vi "XY stage Buttons (reduced).vi"() -> ()   [LabVIEW 2017]
panel:
  in  "Move Inverse":bool
  in  "Move Normal":bool
  out "Expected Output":cluster{"X":dbl, "Y":dbl}[](graph)
  out "Total Time Horizontal":dbl
  out "Total Time Vertical":dbl
  in  "Velocity and Acceleration of Absolute":cluster{"Velocity":dbl, "Acceleration":dbl}={"Velocity"=150.0, "Acceleration"=2000.0} {"Acceleration" min=0.0; "Velocity" min=0.0}
  in  "Abort Motion":bool
  out "Total Y Path":dbl
  in  "Absolute Movement 2":cluster{"X Position":dbl, "Y Position":dbl}[](array[cluster]) {"Y Position" min=-100.0 max=100.0; "X Position" min=-100.0 max=100.0}
  in  "Start Absolute 2":bool
  out "Current Y Position":dbl[](array[numeric])
  out "Current X Position":dbl[](array[numeric])
  out "Total X Path":dbl
  in  "Number of Horizontal Segments":u32
  in  "Number of Vertical Segments":u32
  in  "Horizontal Segments Parameters":T1(array[cluster]) {"velocity" min=0.0; "Y rel dist" min=-100.0 max=100.0; "X rel dist" min=-100.0 max=100.0}
  in  "Vertical Segments Parameters":T1(array[cluster]) {"velocity" min=0.0; "Y rel dist" min=-100.0 max=100.0; "X rel dist" min=-100.0 max=100.0}
  in  "Absolute Movement 1":cluster{"X Position":dbl, "Y Position":dbl}[](array[cluster]) {"Y Position" min=-100.0 max=100.0; "X Position" min=-100.0 max=100.0}
  in  "Start Absolute 1":bool
  in  "Go Home":bool
  in  "Kill All":bool
  # "Relative Movement"
  # "Absolute Movement"
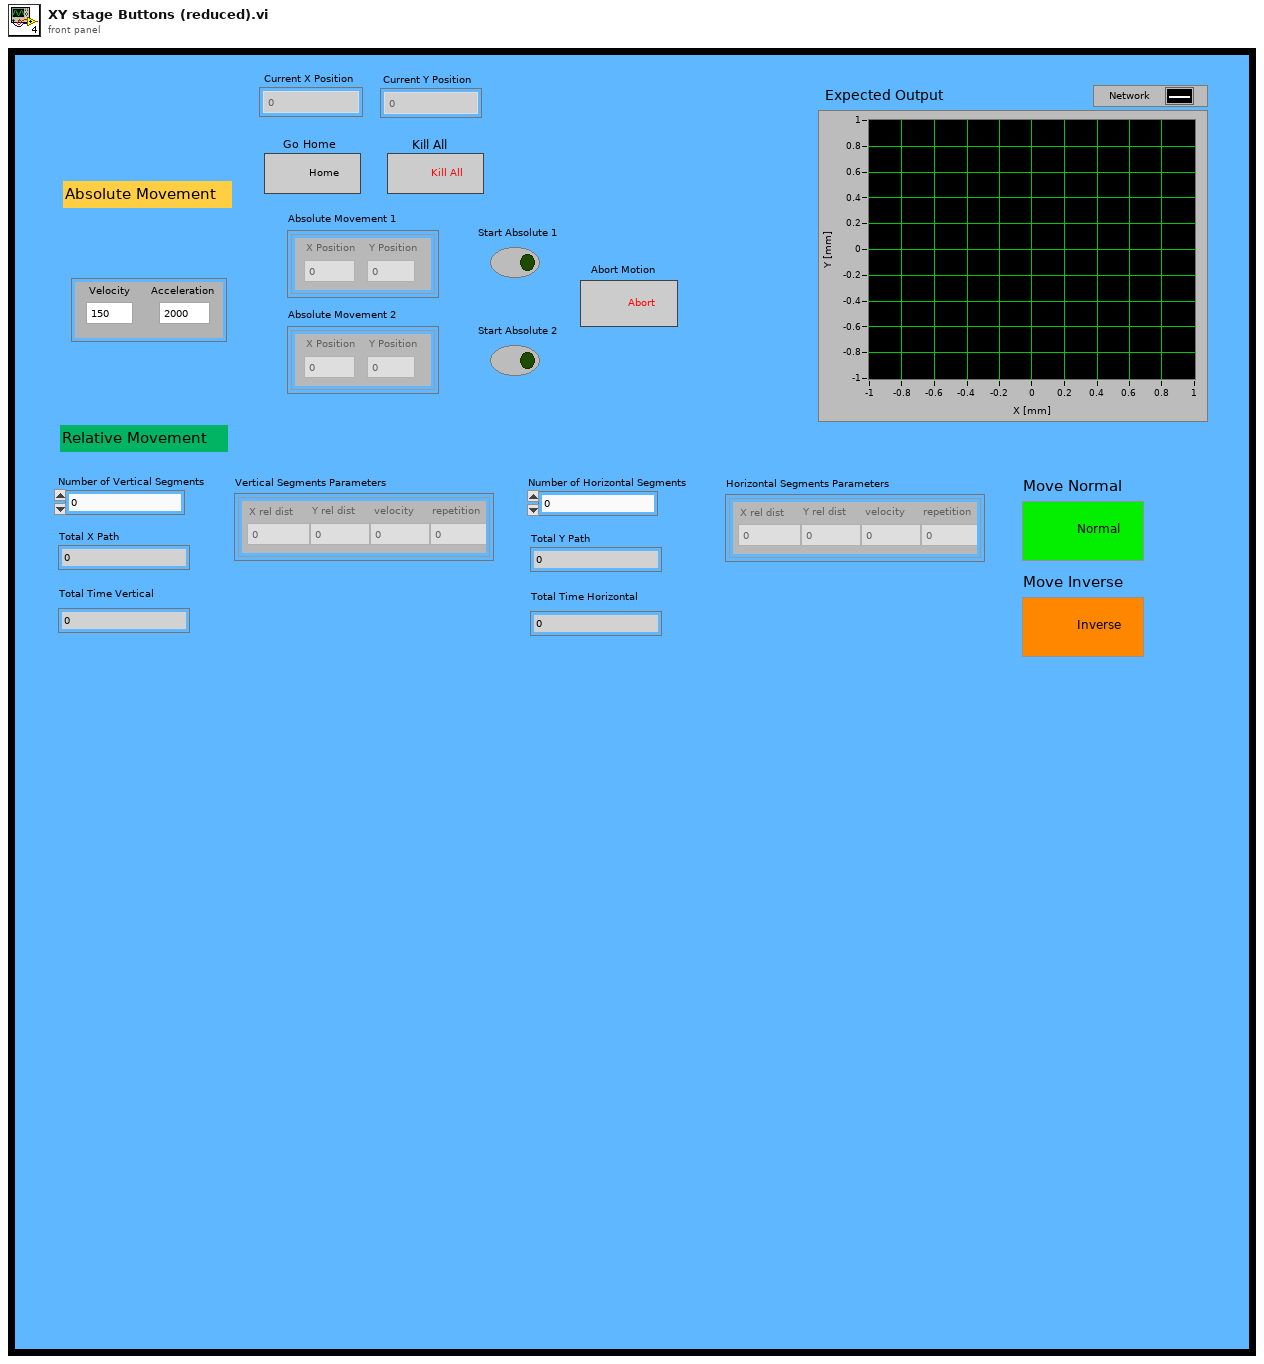
[diagram p1: front panel]
types:
  T1 = cluster{"X rel dist":dbl, "Y rel dist":dbl, "velocity":dbl, "repetition":u32}[]
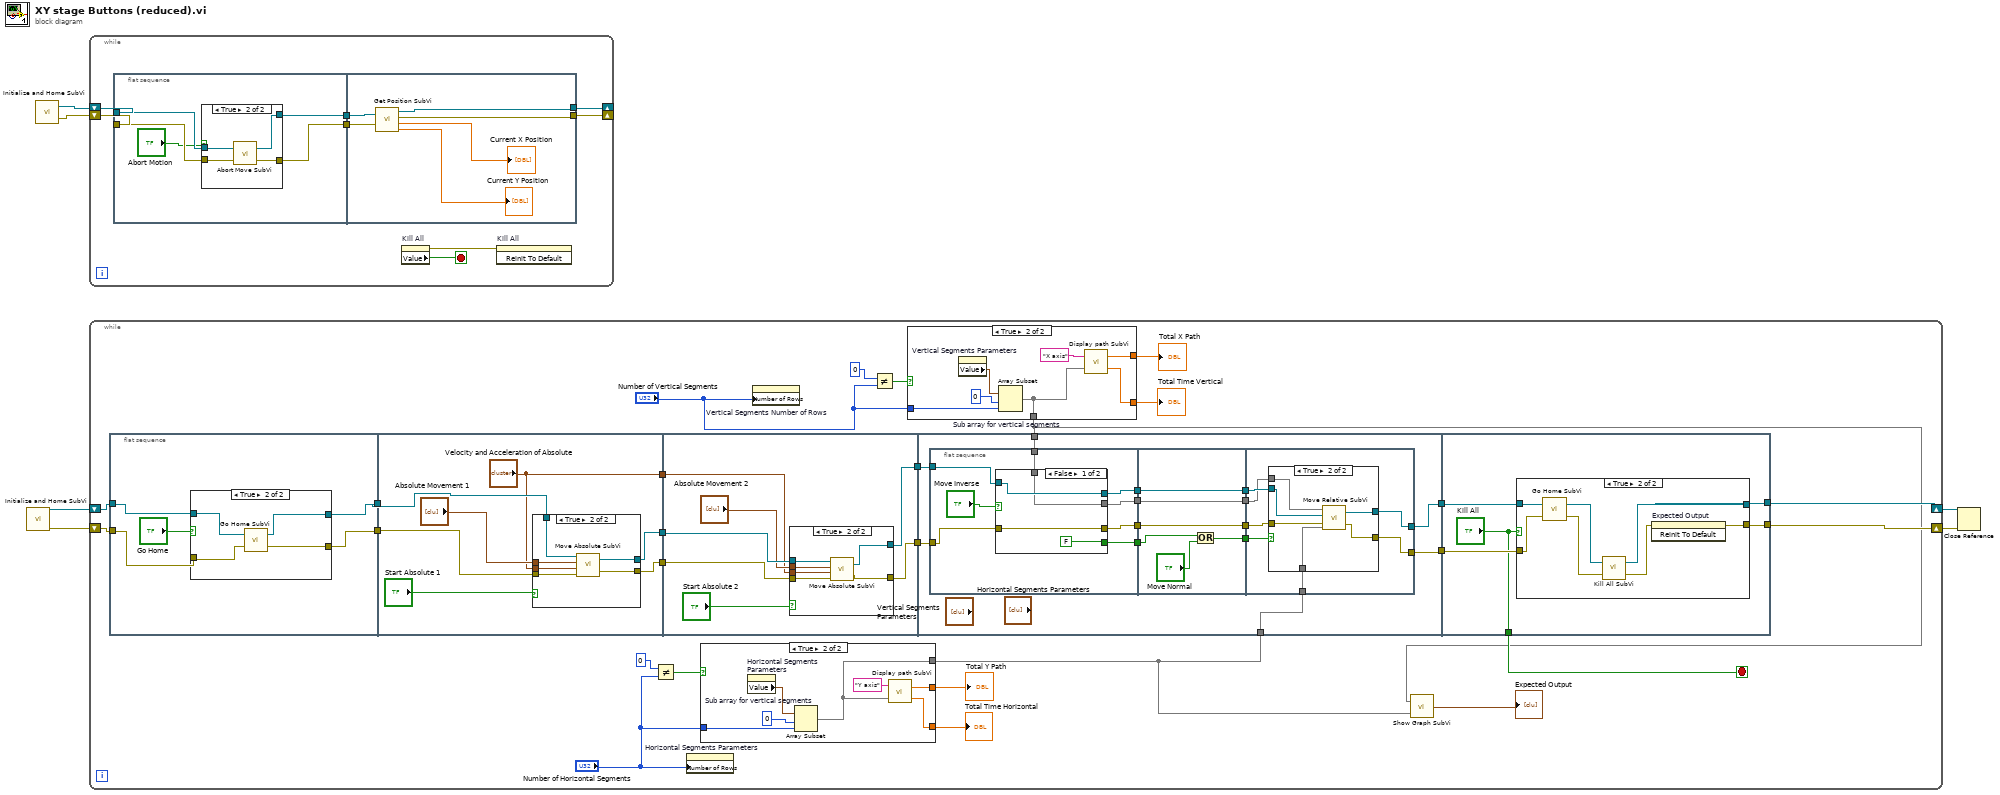
[diagram p0: block diagram]
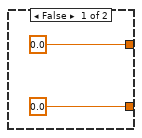
[diagram p2: hidden frame]
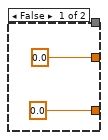
[diagram p3: hidden frame]
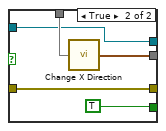
[diagram p7: hidden frame]
diagram:
  n1 = call "Initialize and Home SubVi.vi"() -> ("error out"=w5:errorcluster, "reference out"=w6:refnum<k24>)  [unwired: 2 in]
  n2 = call "Initialize and Home SubVi.vi"() -> ("error out"=w2:errorcluster, "reference out"=w3:refnum<k24>)  [unwired: 2 in]
  n3 = while {
    shift-right: [w14] -> _
    shift-left: w3 -> [w12]
    shift-right: [w13] -> _
    shift-left: w2 -> [w11]
    stop <- w8 stop-if-true
    n4 = flat-sequence {
      tunnel: w11 -> [w17]
      tunnel: w12 -> [w18]
      tunnel: [w19] -> w10
      tunnel: [w16] -> w9
      tunnel: [w31] -> w14
      tunnel: [w30] -> w13
      tunnel: w10 -> [w27]
      tunnel: w9 -> [w26]
      frame #0 {
        n5 = case shown="True" "Abort Motion" {
          tunnel: [w21 w24] -> w19
          tunnel: w18 -> [w21 w25]
          tunnel: w17 -> [w20 w23]
          tunnel: [w20 w22] -> w16
          frame False {
          }
          frame True {
            n6 = call "Abort Move SubVi.vi"("error in"=w23, "reference in"=w25) -> ("error out"=w22:errorcluster, "reference out"=w24:refnum<k24>)
          }
        }
      }
      frame #1 {
        n7 = call "Get Position SubVi.vi"("reference in"=w27, "error in"=w26) -> ("reference out"=w31:refnum<k24>, "error out"=w30:errorcluster, "Current X Position"=→"Current X Position":dbl[], "Current Y Position"=→"Current Y Position":dbl[])
      }
    }
    n8 = property on="Kill All" class="Bool (strict)"() -> (error out=w7:errorcluster, "Value"=w8:bool)  [unwired: 2 in, 1 out]
    n9 = invoke on="Kill All" class="Bool (strict)" method="Reinit To Default"(error in=w7) -> ()  [unwired: 2 in, 3 out]
  }
  n10 = while {
    shift-right: [w46] -> w4
    shift-left: w6 -> [w58]
    shift-right: [w45] -> w1
    shift-left: w5 -> [w57]
    stop <- w54 stop-if-true
    n11 = flat-sequence {
      tunnel: w58 -> [w77]
      tunnel: [w78] -> w56
      tunnel: w57 -> [w80]
      tunnel: [w81] -> w55
      tunnel: w56 -> [w94]
      tunnel: w55 -> [w92]
      tunnel: [w90] -> w53
      tunnel: [w89] -> w51
      tunnel: ["Velocity and Acceleration of Absolute"] -> w47
      tunnel: w53 -> [w106]
      tunnel: [w107] -> w52
      tunnel: w51 -> [w109]
      tunnel: [w108] -> w50
      tunnel: w47 -> [w104]
      tunnel: [w120] -> w49
      tunnel: w52 -> [w130]
      tunnel: [w121] -> w48
      tunnel: w50 -> [w129]
      tunnel: w43 -> [w131]
      tunnel: w32 -> [w122]
      tunnel: ["Kill All"] -> w54
      tunnel: w48 -> [w173]
      tunnel: w49 -> [w174]
      tunnel: [w172] -> w46
      tunnel: [w171] -> w45
      frame #0 {
        n12 = case shown="True" "Go Home" {
          tunnel: [w82 w87] -> w81
          tunnel: w80 -> [w82 w86]
          tunnel: [w83 w85] -> w78
          tunnel: w77 -> [w83 w84]
          frame False {
          }
          frame True {
            n13 = call "Go Home SubVi.vi"("error in"=w86, "reference in"=w84) -> ("error out"=w87:errorcluster, "reference out"=w85:refnum<k24>)
          }
        }
      }
      frame #1 {
        n14 = case shown="True" "Start Absolute 1" {
          tunnel: w94 -> [w95 w102]
          tunnel: "Absolute Movement 1" -> [_ w101]
          tunnel: w92 -> [w96 w100]
          tunnel: "Velocity and Acceleration of Absolute" -> [_ w99]
          tunnel: [w95 w98] -> w90
          tunnel: [w96 w97] -> w89
          frame False {
          }
          frame True {
            n15 = call "Move Absolute SubVi.vi"("error in"=w100, "Vel and Acc"=w99, "Absolute Movement"=w101, "reference in"=w102) -> ("error out"=w97:errorcluster, "reference out"=w98:refnum<k24>)
          }
        }
      }
      frame #2 {
        n16 = case shown="True" "Start Absolute 2" {
          tunnel: w109 -> [w110 w117]
          tunnel: [w110 w116] -> w108
          tunnel: [w111 w115] -> w107
          tunnel: w106 -> [w111 w114]
          tunnel: "Absolute Movement 2" -> [_ w113]
          tunnel: w104 -> [_ w112]
          frame False {
          }
          frame True {
            n17 = call "Move Absolute SubVi.vi"("error in"=w117, "Vel and Acc"=w112, "Absolute Movement"=w113, "reference in"=w114) -> ("error out"=w116:errorcluster, "reference out"=w115:refnum<k24>)
          }
        }
      }
      frame #3 {
        n18 = flat-sequence {
          tunnel: w131 -> [w133]
          tunnel: w130 -> [w137]
          tunnel: w129 -> [w135]
          tunnel: [w139] -> w128
          tunnel: [w136] -> w127
          tunnel: [w134] -> w126
          tunnel: [w132] -> w119
          tunnel: w128 -> [w154]
          tunnel: w127 -> [w153]
          tunnel: w126 -> [w152]
          tunnel: [w154] -> w125
          tunnel: [w153] -> w124
          tunnel: [w152] -> w123
          tunnel: w119 -> [w151]
          tunnel: [w149] -> w118
          tunnel: w125 -> [w159]
          tunnel: w124 -> [w161]
          tunnel: w123 -> [w160]
          tunnel: w122 -> [w158]
          tunnel: [w157] -> w121
          tunnel: [w156] -> w120
          tunnel: w118 -> [w155]
          frame #0 {
            n19 = case shown="False" "Move Inverse" {
              tunnel: [w140 w148] -> w139
              tunnel: [FALSE TRUE] -> w132
              tunnel: w133 -> [w140 w146]
              tunnel: w137 -> [w143 w145]
              tunnel: [w143 w145] -> w136
              tunnel: w135 -> [w142 w144]
              tunnel: [w142 w144] -> w134
              frame False {
              }
              frame True {
                n20 = call "Change X Direction.vi"("Vertical Segments Parameters in"=w146) -> ("Vertical Segments Parameters out"=w148:T1)
              }
            }
          }
          frame #1 {
            n21 = Or(x=w151, y="Move Normal") -> (x .or. y?=w149:bool)
          }
          frame #2 {
            n22 = case shown="True" w155 {
              tunnel: w161 -> [w163 w169]
              tunnel: w160 -> [w162 w165]
              tunnel: [w162 w164] -> w157
              tunnel: [w163 w166] -> w156
              tunnel: w159 -> [_ w167]
              tunnel: w158 -> [_ w168]
              frame False {
              }
              frame True {
                n23 = call "Move Relative SubVi.vi"("Horizontal Segments Parameters"=w168, "error in"=w165, "reference in"=w169, "Vertical Segments Parameters"=w167) -> ("error in 2"=w164:errorcluster, "reference out"=w166:refnum<k24>)
              }
            }
          }
        }
      }
      frame #4 {
        n24 = case shown="True" "Kill All" {
          tunnel: w174 -> [w176 w180]
          tunnel: w173 -> [w175 w178]
          tunnel: [w176 w183] -> w172
          tunnel: [w175 w181] -> w171
          frame False {
          }
          frame True {
            n25 = call "Go Home SubVi.vi"("error in"=w178, "reference in"=w180) -> ("error out"=w177:errorcluster, "reference out"=w179:refnum<k24>)
            n26 = call "Kill All SubVi.vi"("error in"=w177, "reference in"=w179) -> ("error out"=w182:errorcluster, "reference out"=w183:refnum<k24>)
            n27 = invoke on="Expected Output" class="XYGraph (strict)" method="Reinit To Default"(error in=w182) -> (error out=w181:errorcluster)  [unwired: 2 in, 2 out]
          }
        }
      }
    }
    n28 = Not Equal?(x=0, y="Number of Horizontal Segments") -> (x != y?=w38:bool)
    n29 = property on="Horizontal Segments Parameters" class="Arr (strict)"("Number of Rows"="Number of Horizontal Segments") -> ()  [unwired: 2 in, 2 out]
    n30 = case shown="True" w38 {
      tunnel: [_ w74] -> w32
      tunnel: "Number of Horizontal Segments" -> [_ w73]
      tunnel: [0.0 ("Total Time") w70] -> w36
      tunnel: [0.0 ("Total Path") w71] -> w35
      frame False {
      }
      frame True {
        n31 = property on="Horizontal Segments Parameters" class="Arr (strict)"() -> ("Value"=w75:T1)  [unwired: 2 in, 2 out]
        n32 = Array Subset "Sub array for vertical segments"(array=w75, index=0, length=w73) -> (w74:T1)
        n33 = call "Display path SubVi.vi"("Array"=w74, "Combo Box"="Y axis") -> ("Total Time"=w70:dbl, "Total Path"=w71:dbl)
      }
    }
    "Total Y Path" <- w35
    "Total Time Horizontal" <- w36
    n34 = property on="Vertical Segments Number of Rows" class="Arr (strict)"("Number of Rows"="Number of Vertical Segments") -> ()  [unwired: 2 in, 2 out]
    n35 = Not Equal?(x=u32 0, y="Number of Vertical Segments") -> (x != y?=w37:bool)
    n36 = case shown="True" w37 {
      tunnel: [_ w65] -> w43
      tunnel: "Number of Vertical Segments" -> [_ w64]
      tunnel: [0.0 ("Total Path") w62] -> w34
      tunnel: [0.0 ("Total Time") w61] -> w33
      frame False {
      }
      frame True {
        n37 = property on="Vertical Segments Parameters" class="Arr (strict)"() -> ("Value"=w66:T1)  [unwired: 2 in, 2 out]
        n38 = Array Subset "Sub array for vertical segments"(array=w66, index=0, length=w64) -> (w65:T1)
        n39 = call "Display path SubVi.vi"("Array"=w65, "Combo Box"="X axis") -> ("Total Time"=w61:dbl, "Total Path"=w62:dbl)
      }
    }
    "Total X Path" <- w34
    "Total Time Vertical" <- w33
    n40 = call "Show Graph SubVi.vi"("Horizontal Segments Parameters"=w32, "Vertical Segments Parameters"=w43) -> ("Output Array"=→"Expected Output":cluster{"X":dbl, "Y":dbl}[])
  }
  n41 = Close Reference(reference=w4, error in (no error)=w1) -> ()  [unwired: 1 out]
